vi "close.vi"(8 "error in":errorcluster, 11 "Handle":i32) -> (0 "error out":errorcluster)   [LabVIEW 2025, in "LabJackEKG.lvlib"]
uses:
  LabJackEKG.lvlib
panel:
  # "LabJack V0.10\nClose"
  # "09.05.2025"
  # "Blaz Kelbl"
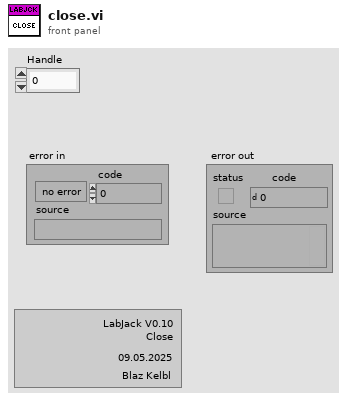
[diagram p1: front panel]
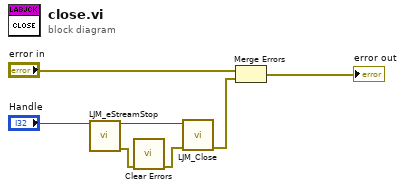
[diagram p0: block diagram]
diagram:
  n1 = call <vilib>:"LJM_eStreamStop.vi"("Handle In"="Handle") -> ("Handle Out"=w2:i32, "error out"=w1:errorcluster)  [unwired: 13 in]
  n2 = call <vilib>:"Clear Errors.vi"("error in (no error)"=w1) -> ("error out"=w4:errorcluster)  [unwired: 5 in, 1 out]
  n3 = call <vilib>:"LJM_Close.vi"("error in"=w4, "Handle"=w2) -> ("error out"=w7:errorcluster)  [unwired: 9 in]
  n4 = Merge Errors("error in", w7) -> (→"error out":errorcluster)
